vi "Scan Start Measurement Command Response.vi"(3 "Error In (No Error)":errorcluster, 4 "Measurement Type In (Normal)":i32(ring) items=["Normal", "Concurrent", "Continuous"], 5 "Measurement Response":string) -> (0 "Error Out":errorcluster, 1 "Number of Measurements":i32, 2 "Max Acquisition Time":i32)   [LabVIEW 2016, in "SDI-12.lvlib"]
doc: "Scans SDI-12 Start Measurement Command Response from Normal and Concurrent Measurements, and obtains the maximum sensor acquisition time and total number of measurements that the sensor will return.\n\nNOTE: Continuous Measurements commands only reply with data. Please use the Scan Send Data Command Response VI for Continuous Measurements.\n\nExpected Response:\n\nNormal Measurement atttn<CR><LF>\nConcurrent Measurement atttnn<CR><LF>\n\n\na = the sensor address\nttt = the specified time, in seconds, until the sensor will have the measurement(s) ready\nn/nn =total measurements that the sensor will make"
uses:
  SDI-12.lvlib
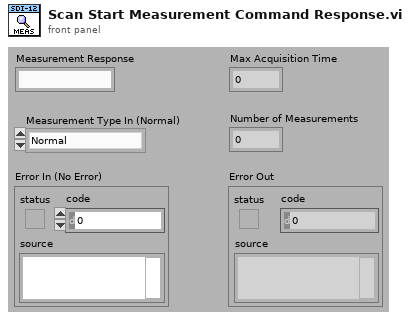
[diagram p1: front panel]
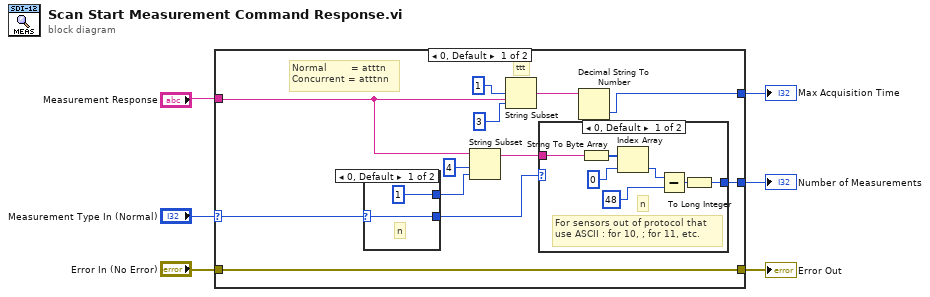
[diagram p0: block diagram]
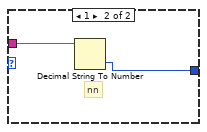
[diagram p2: hidden frame]
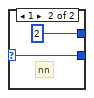
[diagram p3: hidden frame]
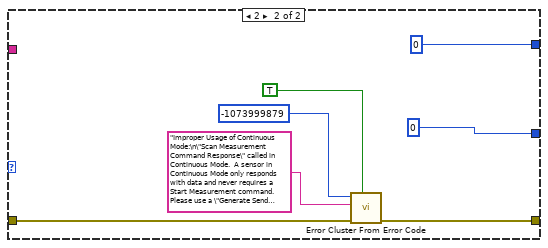
[diagram p4: hidden frame]
diagram:
  n1 = case shown="0, Default" "Measurement Type In (Normal)" {
    selector: "Measurement Type In (Normal)" -> [w8 _]
    tunnel: [w13 0] -> w6
    tunnel: [w9 0] -> w5
    tunnel: "Measurement Response" -> [w12 _]
    tunnel: "Error In (No Error)" -> [w11 w37]
    tunnel: [w11 w34] -> w1
    frame 0, Default {
      # "Normal        = atttn\nConcurrent = atttnn"
      # "ttt"
      n2 = case shown="0, Default" w8 {
        selector: w8 -> [w28 w30]
        tunnel: [1 ("length (rest)") 2 ("length (rest)")] -> w17
        tunnel: [w28 w30] -> w7
        frame 0, Default {
          # "n"
        }
        frame 1 {
          # "nn"
        }
      }
      n3 = String Subset(string=w12, offset (0)=4 ("length (rest)"), length (rest)=w17) -> (substring=w10:string)
      n4 = String Subset(string=w12, offset (0)=1, length (rest)=3 ("length (rest)")) -> (substring=w18:string)
      n5 = case shown="0, Default" w7 {
        tunnel: w10 -> [w25 w27]
        tunnel: [w19 w26] -> w9
        frame 0, Default {
          # "For sensors out of protocol that\nuse ASCII : for 10, ; for 11, etc."
          # "n"
          n6 = String To Byte Array(string=w25) -> (unsigned byte array=w24:u8[])
          n7 = Index Array(array=w24, index=0) -> (element=w22:u8)
          n8 = Subtract(x=w22, y=u8 48) -> (x-y=w20:u8)
          n9 = To Long Integer(number=w20) -> (32bit integer=w19:i32)
        }
        frame 1 {
          # "nn"
          n10 = Decimal String To Number(string=w27) -> (number=w26:i32)  [unwired: 2 in, 1 out]
        }
      }
      n11 = Decimal String To Number(string=w18) -> (number=w13:i32)  [unwired: 2 in, 1 out]
    }
    frame 2 {
      n12 = call <vilib>:"Error Cluster From Error Code.vi"("show call chain? (False)"=TRUE, "error in (no error)"=w37, "error message (\"\")"="Improper Usage of Continuous Mode:\n\"Scan Measurement Command Response\" called in Continuous Mode.  A sensor in Continuous Mode only responds with data and never requires a Start Measurement command.  Please use a \"Generate Send Command\" followed by a \"Send Data Command Response\" to gather the data obtained by a Continuous Mode sensor.  " ("error message (\"\")"), "error code (0)"=-1073999879 ("error code")) -> ("error out"=w34:errorcluster)  [unwired: 5 in]
    }
  }
  "Error Out" <- w1
  "Number of Measurements" <- w5
  "Max Acquisition Time" <- w6
